vi "startBroadcastSetForceFrame.vi"(0 "FAILC in":refnum<class "FAILC.lvclass">, 5 "ModbusBuffer in":refnum<class "ModbusBuffer.lvclass">, 7 "BroadcastCounter":u8, 9 "SlewFlag":bool, 11 "error in (no error)":errorcluster) -> (4 "FAILC out":refnum<class "FAILC.lvclass">, 6 "ModbusBuffer out":refnum<class "ModbusBuffer.lvclass">, 15 "error out":errorcluster)   [LabVIEW 2016, in "RTFAILC.lvlib" / "FAILC.lvclass"]
uses:
  FAILC.lvclass
  D:/Code/ts_M1M3Support/Common_RT_ILC/ILC/ILC.lvclass
  Common_RT_Modbus/ModbusBuffer/ModbusBuffer.lvclass
  Common_RT_ILC/ILC/ILC.lvclass/ILC.ctl
  Common_RT_Modbus/ModbusBuffer/ModbusBuffer.lvclass/ModbusBuffer.ctl
  Common_RT_Modbus/ModbusBuffer/writeByteInstruction.vi
  Common_RT_ILC/ILC/ILC.lvclass
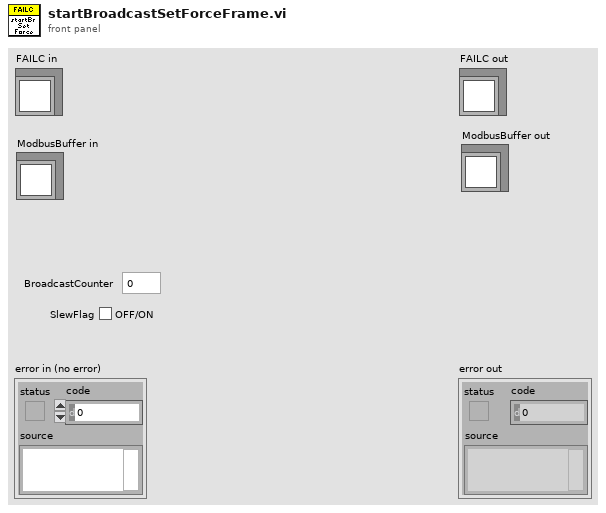
[diagram p1: front panel]
types:
  T1 = typedef "RTILC.lvlib/ILCData.ctl" = cluster{"Constants":T2, "Command":T3, "Telemetry":T5, "Responses":T6, "Timestamps":T8, "Timings":T9}
  T2 = typedef "RTILC.lvlib/ILCConstants.ctl" = cluster{"Subnet":u8, "Address":u8}
  T3 = typedef "RTILC.lvlib/ILCCommand.ctl" = cluster{"Mode":u16, "TemporaryAddress":u8, "ADCScanRate":T4, "ADCChannel":u8, "ADCOffset":sgl, "ADCSensitivity":sgl}
  T4 = typedef "RTILC.lvlib/ILCScanRates.ctl" = u8
  T5 = typedef "RTILC.lvlib/ILCTelemetry.ctl" = cluster{"UniqueID":u64, "FirmwareType":u8, "NetworkNodeType":u8, "ILCOption":u8, "NetworkNodeOption":u8, "MajorRevision":u8, "MinorRevision":u8, "FirmwareName":string, "Mode":u16, "MajorFault":bool, "MinorFault":bool, "FaultOverride":bool, "MainCalibrationError":bool, "BackupCalibrationError":bool, "UniqueIDCRCMismatch":bool, "AppTypeNodeTypeMismatch":bool, "AppMissing":bool, "AppCRCMismatch":bool, "TEDSNotFound":bool, "TEDS1Mismatch":bool, "TEDS2Mismatch":bool, "WatchdogResetDetected":bool, "BrownoutDetected":bool, "EventTrapResetDetected":bool, "MotorPowerFault":bool, "SSRPowerFault":bool, "AuxPowerFault":bool, "SMCPowerFault":bool, "TemporaryAddress":u8, "ADCScanRate":T4, "MainADCCalibrationK":sgl[], "MainSensorOffset":sgl[], "MainSensorSensitivity":sgl[], "BackupADCCalibrationK":sgl[], "BackupSensorOffset":sgl[], "BackupSensorSensitivity":sgl[]}
  T6 = typedef "RTILC.lvlib/ILCResponses.ctl" = cluster{"ReportServerID":T7, "ReportServerStatus":T7, "Mode":T7, "TemporaryAddress":T7, "Reset":T7, "ADCScanRate":T7, "ADCOffsetSensitivity":T7, "ReportCalibrationData":T7}
  T7 = typedef "RTModbus.lvlib/ExceptionCodes.ctl" = u16
  T8 = typedef "RTILC.lvlib/ILCTimestamps.ctl" = cluster{"ReportServerID":dbl, "ReportServerStatus":dbl, "Mode":dbl, "TemporaryAddress":dbl, "Reset":dbl, "ADCScanRate":dbl, "ADCOffsetSensitivity":dbl, "ReportCalibrationData":dbl}
  T9 = typedef "RTILC.lvlib/ILCTimings.ctl" = cluster{"ReportServerID":u32, "ReportServerStatus":u32, "Mode":u32, "TemporaryAddress":u32, "Reset":u32, "ADCScanRate":u32, "ADCOffsetSensitivity":u32, "ReportCalibrationData":u32}
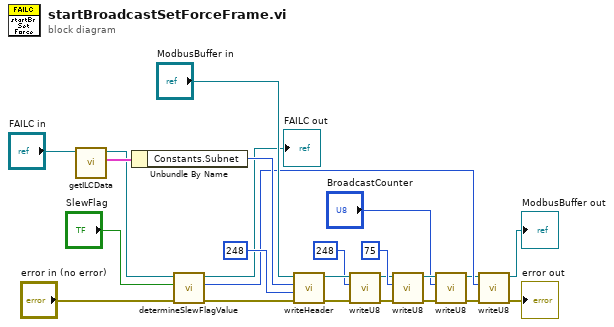
[diagram p0: block diagram]
diagram:
  n1 = call "getILCData.vi"("ILC in"="FAILC in") -> ("ILCData"=w17:T1, "ILC out"=w13:refnum<class "FAILC.lvclass">)  [unwired: 9 in]
  n2 = Unbundle By Name(w17) -> ("Constants.Subnet"=w16:u8)
  n3 = call "determineSlewFlagValue.vi"("error in (no error)"="error in (no error)", "SlewFlag"="SlewFlag", "FAILC in"=w13) -> ("error out"=w7:errorcluster, "FlagValue"=w11:u8, "FAILC out"=→"FAILC out":refnum<class "FAILC.lvclass">)  [unwired: 6 in]
  n4 = call "writeHeader.vi"("error in (no error)"=w7, "Length"=u16 248, "Subnet"=w16, "ModbusBuffer in"="ModbusBuffer in") -> ("error out"=w21:errorcluster, "ModbusBuffer out"=w23:refnum<class "ModbusBuffer.lvclass">)  [unwired: 6 in]
  n5 = call "writeU8.vi"("error in (no error)"=w21, "Input"=u8 248, "ModbusBuffer in"=w23) -> ("error out"=w20:errorcluster, "ModbusBuffer out"=w14:refnum<class "ModbusBuffer.lvclass">)  [unwired: 7 in]
  n6 = call "writeU8.vi"("error in (no error)"=w20, "Input"=u8 75 ("Function"), "ModbusBuffer in"=w14) -> ("error out"=w3:errorcluster, "ModbusBuffer out"=w4:refnum<class "ModbusBuffer.lvclass">)  [unwired: 7 in]
  n7 = call "writeU8.vi"("error in (no error)"=w3, "Input"="BroadcastCounter", "ModbusBuffer in"=w4) -> ("error out"=w1:errorcluster, "ModbusBuffer out"=w5:refnum<class "ModbusBuffer.lvclass">)  [unwired: 7 in]
  n8 = call "writeU8.vi"("error in (no error)"=w1, "Input"=w11, "ModbusBuffer in"=w5) -> ("error out"=→"error out":errorcluster, "ModbusBuffer out"=→"ModbusBuffer out":refnum<class "ModbusBuffer.lvclass">)  [unwired: 7 in]
